vi "Write Image Delays.vi"(8 "error in (no error)":errorcluster, 10 "Image Delays":string[](array[string]), 11 "Header Contents in":refnum<class "Header Contents.lvclass">) -> (0 "error out":errorcluster, 3 "Header Contents out":refnum<class "Header Contents.lvclass">)   [LabVIEW 2018, in "Header Contents.lvclass"]
uses:
  Header Contents.lvclass
  Header Contents.lvclass/Header Contents.ctl
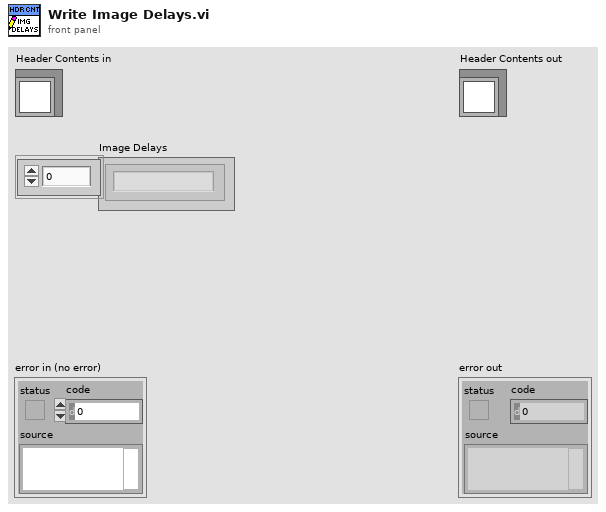
[diagram p1: front panel]
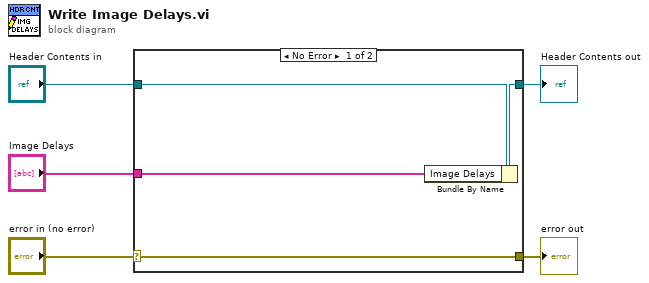
[diagram p0: block diagram]
diagram:
  n1 = case shown="No Error" "error in (no error)" {
    selector: "error in (no error)" -> [w9 w10]
    tunnel: [w9 w10] -> w4
    tunnel: [w7 w11] -> w2
    tunnel: "Header Contents in" -> [w8 w11]
    tunnel: "Image Delays" -> [w6 _]
    frame No Error {
      n2 = Bundle By Name(cluster=w8, "Image Delays"=w6) -> (w7:refnum<class "Header Contents.lvclass">)
    }
    frame Error {
    }
  }
  "error out" <- w4
  "Header Contents out" <- w2
